vi "reset_k7_link.vi"(8 "error in (no error)":errorcluster, 11 "address":string="10.3.173.11") -> (0 "error out":errorcluster)   [LabVIEW 2017]
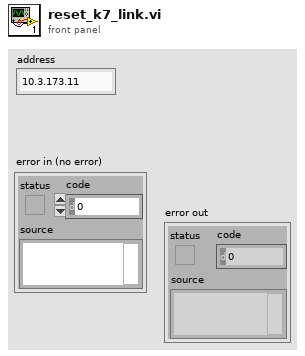
[diagram p1: front panel]
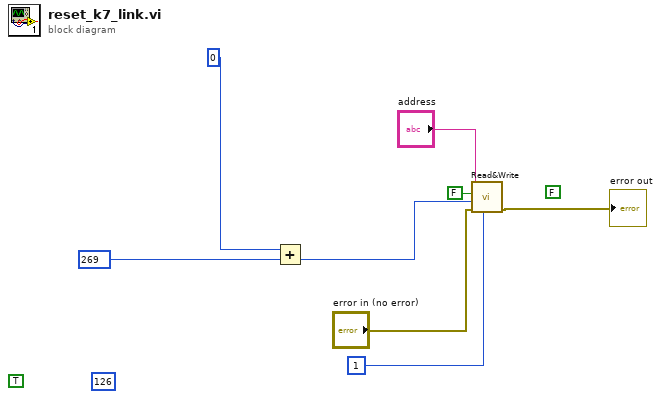
[diagram p0: block diagram]
diagram:
  (unwired) FALSE ("Read (TRUE)")
  (unwired) u8 126 ("In 3")
  (unwired) TRUE
  n1 = Add(x=0, y=u32 269 ("Address")) -> (x+y=w3:u32)
  n2 = call "Read&Write.vi"("In"=u8 1, "error in (no error)"="error in (no error)", "Address"=w3, "Read (TRUE)"=FALSE, "address"="address") -> ("error out"=→"error out":errorcluster)  [unwired: 5 in, 1 out]
